vi "PV Digiline adjustment.vi"(8 "error in (no error)":errorcluster, 9 "Digiline adjustment - Cluster":T1 {"Switch Filament HPT200" items=["Filament auto (default)", "Filament 1", "Filament 2"]; "Sensor Switch Mode" items=["switch", "trans_Lo", "trans_Hi"]; "Parameter" items=[" DeGas (on/off)  (for HPT only) ", " Sensor (on/off)", " Sensor Switch Mode", " Switch Filament (for HPT200 only)"]}, 10 "Adress of unit":u16=1 max=999 step=1, 11 "VISA session":refnum<visa-resource-name>) -> (0 "error out":errorcluster, 2 "response (data)":string, 3 "dup VISA session":refnum<visa-resource-name>)   [LabVIEW 2012, in "Pfeiffer Vacuum.lvlib"]
doc: "There are four parameters available, only one of which can be enabled at a time. \n\n0 - DeGas [off/on] (default) - for HPT only - Para 040\n1 - Filament HPT or CC Sensor MPT [off/on] - Para 041\n2 - Sensor Switch Mode - Para 049\n3 - Switch Filament (for HPT200 only) - Para 022\n\nNote: The three controls right of this one will set the appropriate values for the selected parameter. Any settings for an parameter that is not selected will be ignored. If a value is out of range, it will be changed to either the upper or the lower limit of the range.\n\nTo use one of the operations after you have configured it, use the read measurement VI, not the Example VI. The example VI will disable any math operation in effect."
uses:
  <instrlib>/Pfeiffer Vacuum/Pfeiffer Vacuum.lvlib
  <instrlib>/Pfeiffer Vacuum/Public/DigiLine/DigiLine adjustment - Cluster.ctl
panel:
  # "<-------          ------->     \n DeGas (on/off)   :       off                   on             \n Sensor (on/off)  :       off                   on"
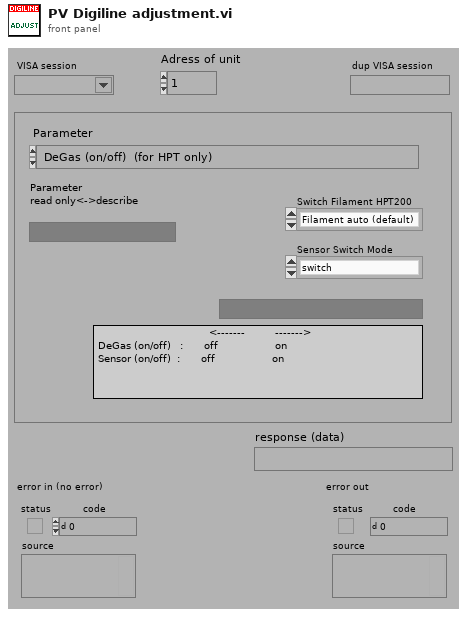
[diagram p1: front panel]
types:
  T1 = typedef "Pfeiffer Vacuum.lvlib/DigiLine adjustment - Cluster.ctl" = cluster{"Parameter":u16, "Parameter\nread only<->describe":bool, "off/on":bool, "Sensor Switch Mode":u16, "Switch Filament HPT200":u16}
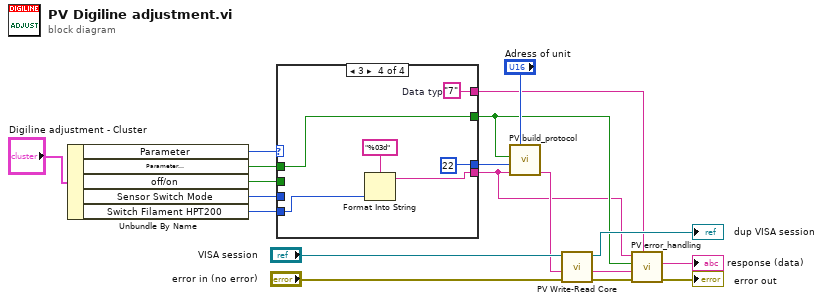
[diagram p0: block diagram]
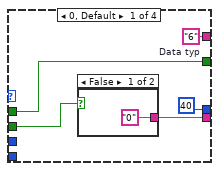
[diagram p2: hidden frame]
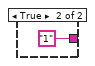
[diagram p3: hidden frame]
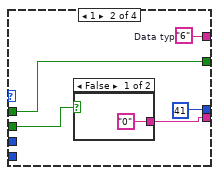
[diagram p4: hidden frame]
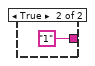
[diagram p5: hidden frame]
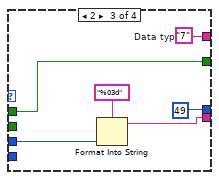
[diagram p6: hidden frame]
diagram:
  n1 = Unbundle By Name("Digiline adjustment - Cluster") -> ("Parameter"=w17:u16, "Parameter\nread only<->describe"=w15:bool, "off/on"=w16:bool, "Sensor Switch Mode"=w3:u16, "Switch Filament HPT200"=w1:u16)
  n2 = case shown="3" w17 {
    tunnel: [u16 40 ("Parameter-number") u16 41 ("Parameter-number") u16 49 ("Parameter-number") u16 22 ("Parameter-number")] -> w18
    tunnel: [w23 w30 w34 w41] -> w7
    tunnel: [w22 w31 w39 w45] -> w8
    tunnel: [w21 w29 w38 w44] -> w6
    tunnel: w16 -> [w20 w27 _ _]
    tunnel: w15 -> [w22 w31 w39 w45]
    tunnel: w3 -> [_ _ w35 _]
    tunnel: w1 -> [_ _ _ w40]
    frame 0, Default {
      w21 = "6"  # Data typ
      n3 = case shown="False" w20 {
        tunnel: ["0" ("Data") "1" ("Data")] -> w23
        frame False {
        }
        frame True {
        }
      }
    }
    frame 1 {
      w29 = "6"  # Data typ
      n4 = case shown="False" w27 {
        tunnel: ["0" ("Data") "1" ("Data")] -> w30
        frame False {
        }
        frame True {
        }
      }
    }
    frame 2 {
      w38 = "7"  # Data typ
      n5 = Format Into String(format string="%03d" ("Format-String"), w35) -> (resulting string=w34:string)  [unwired: 2 in, 1 out]
    }
    frame 3 {
      w44 = "7"  # Data typ
      n6 = Format Into String(format string="%03d" ("Format-String"), w40) -> (resulting string=w41:string)  [unwired: 2 in, 1 out]
    }
  }
  n7 = call <instrlib>:"PV build_protocol.vi"("Data"=w7, "Parameter-number"=w18, "parameter\nread<->describe"=w8, "Adress"="Adress of unit") -> ("output"=w12:string)  [unwired: 3 in]
  n8 = call <instrlib>:"PV Write-Read Core.vi"("error in"="error in (no error)", "Write data in"=w12, "VISA session"="VISA session") -> ("error out"=w9:errorcluster, "response (data) out"=w10:string, "dup VISA session"=→"dup VISA session":refnum<visa-resource-name>)  [unwired: 2 in]
  n9 = call <instrlib>:"PV error_handling.vi"("Data Typ in"=w6, "error in"=w9, "response (data) in"=w10, "Parameter\nread only<->describe"=w8, "data in"=w7) -> ("error out"=→"error out":errorcluster, "Data out"=→"response (data)":string)  [unwired: 4 in, 1 out]
